vi "ProdaNG.Tree.Proc.Update.vi"(4 "Configuration":T1={"ShowUnreleased"=FALSE, "Param1"="", "ParamStartIdx"=0, "Slots"=1} {"Slots" min=1 max=2; "ParamStartIdx" min=0 max=1}, 6 "VariantFilter":string caption="Wabco Part Filter", 7 "Tree":refnum<vi>, 8 "error in (no error)":errorcluster, 11 "dbHandle in":i32) -> (0 "error out":errorcluster, 3 "dbHandle out":i32)   [LabVIEW 2016]
uses:
  ProdaNG.Configurator.Config.ctl
  ProdaNG.Configurator.Glb.vi
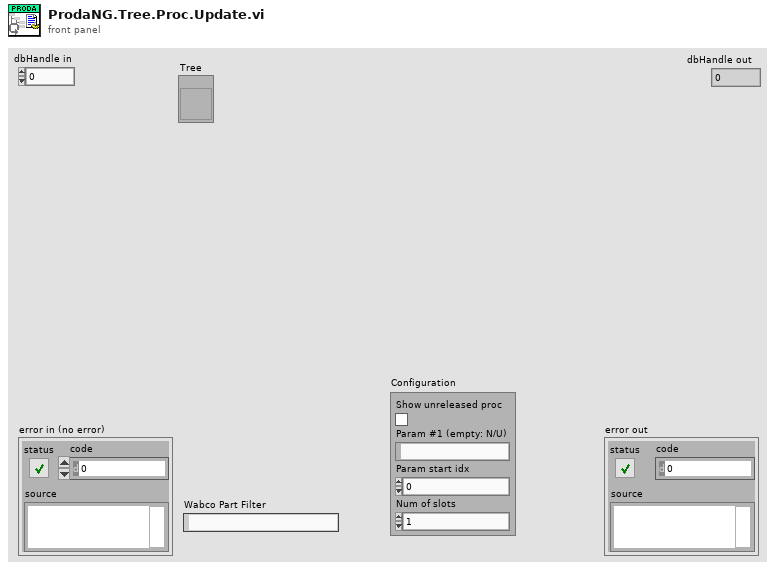
[diagram p1: front panel]
types:
  T1 = typedef "ProdaNG.Configurator.Config.ctl" = cluster{"ShowUnreleased":bool, "Param1":string, "ParamStartIdx":i32, "Slots":i32}
  T2 = cluster{"P_ID":i32, "S_ID":i32, "PS_ID":i32, "WP_ID":i32}
  T3 = typedef "ProdaNG.WabcoPart.ctl" = cluster{"i_id":i32, "workCenterId":i32, "contentId":string, "previewId":string, "mdReason":string, "mdUser":string, "mdTime":string, "productName":string, "wabcoNumber":string}
  T4 = typedef "ProdaNG.Process.ctl" = cluster{"i_id":i32, "productionLineId":i32, "releaseId":i32, "contentId":string, "previewId":string, "mdReason":string, "mdUser":string, "mdTime":string, "description":string}
  T5 = typedef "ProdaNG.ProcessStep.ctl" = cluster{"i_id":i32, "processId":i32, "systemId":i32, "releaseId":i32, "processSequence":i32, "limitYellow":dbl, "limitRed":dbl, "mdReason":string, "mdUser":string, "mdTime":string, "filename":string, "transfer":string, "description":string}
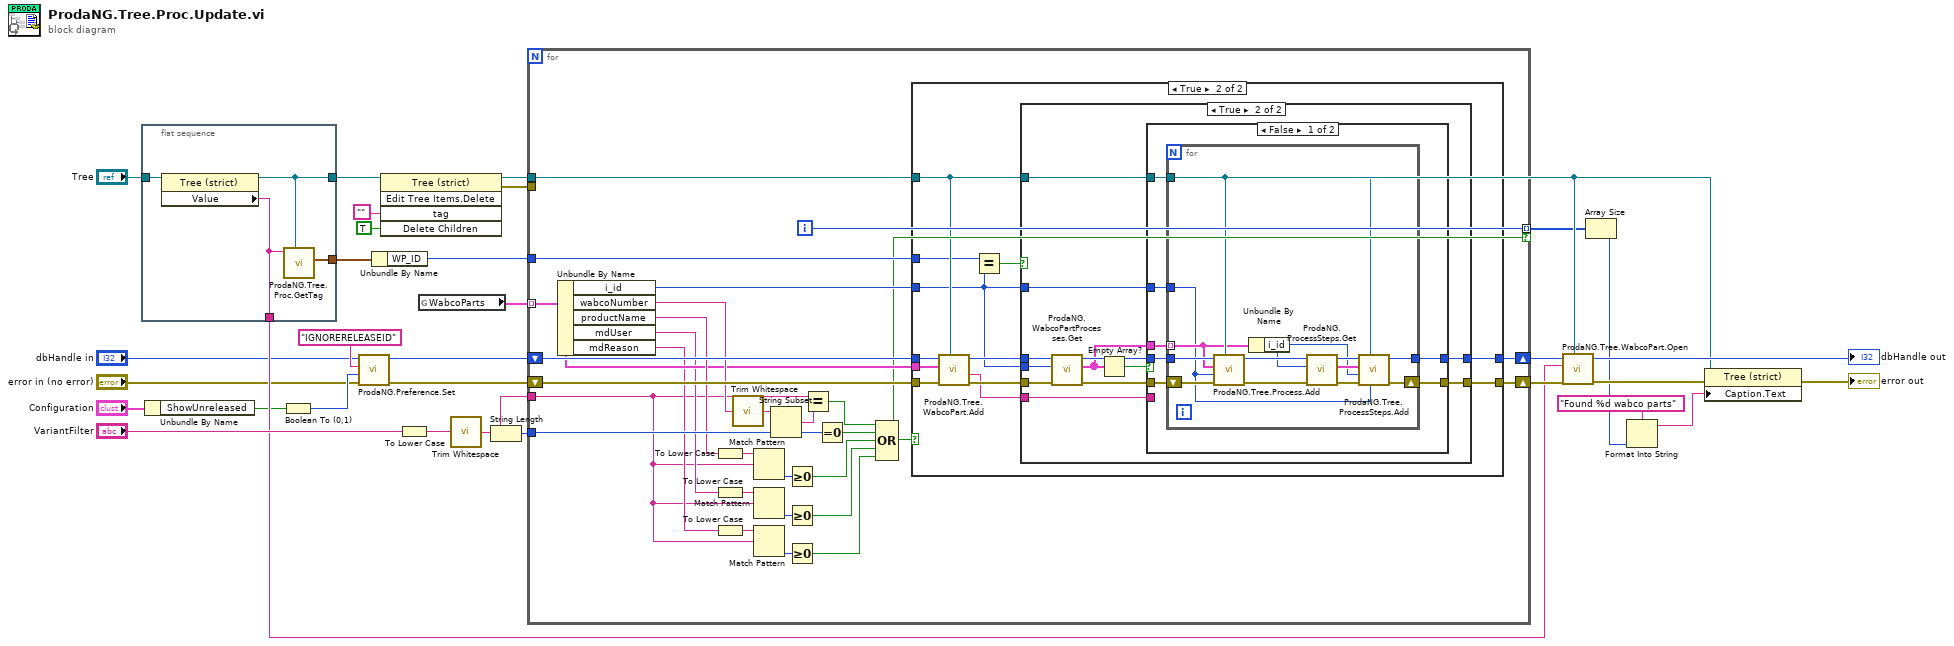
[diagram p0: block diagram]
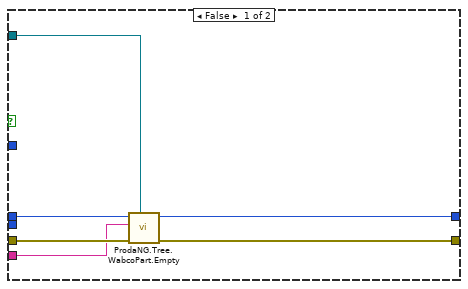
[diagram p3: hidden frame]
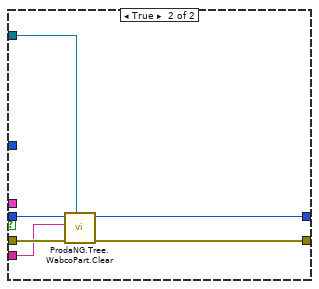
[diagram p4: hidden frame]
diagram:
  n1 = flat-sequence {
    tunnel: "Tree" -> [w34]
    tunnel: [w33] -> w24
    tunnel: [w32] -> w23
    tunnel: [w31] -> w20
    frame #0 {
      n2 = property class="Tree (strict)"(reference=w34) -> (reference out=w33:refnum<vi>, "Value"=w31:string)  [unwired: 1 in, 1 out]
      n3 = call "ProdaNG.Tree.Proc.GetTag.vi"("Tree"=w33, "Tag"=w31) -> ("Identification"=w32:T2)  [unwired: 5 in, 4 out]
    }
  }
  n4 = Unbundle By Name("Configuration") -> ("ShowUnreleased"=w1:bool)
  n5 = Boolean To (0,1)(Boolean=w1) -> (0, 1=w8:i16)
  n6 = call "ProdaNG.Preference.Set.vi"("error in"="error in (no error)", "value"=w8, "key"="IGNORERELEASEID", "dbHandleIn"="dbHandle in") -> ("error out"=w6:errorcluster, "dbHandle"=w5:i32)  [unwired: 6 in]
  n7 = Unbundle By Name(w23) -> ("WP_ID"=w22:i32)
  n8 = invoke class="Tree (strict)" method="Edit Tree Items.Delete"(reference=w24, "tag"="", "Delete Children"=TRUE ("Delete Children?")) -> (reference out=w13:refnum<vi>, error out=w26:errorcluster)  [unwired: 2 in, 3 out]
  n9 = To Lower Case(string="VariantFilter") -> (all lower case string=w17:string)
  n10 = global read "ProdaNG.Configurator.Glb.vi" "WabcoParts"() -> (w16:T3[])
  n11 = call <vilib>:"Trim Whitespace.vi"("string"=w17) -> ("trimmed string"=w18:string)  [unwired: 1 in]
  n12 = String Length(string=w18) -> (length=w19:i32)
  n13 = for {
    shift-right: [w61] -> w30
    shift-left: w5 -> [w62]
    shift-right: [w60] -> w21
    shift-left: w6 -> [w63]
    tunnel: w13 -> [w59]
    tunnel: w26 -> [_]
    tunnel: w22 -> [w58]
    tunnel: w19 -> [w54]
    tunnel: w18 -> [w37]
    tunnel: w16 -> [w49] mode=indexing
    tunnel: [w48] -> w12 mode=indexing if=w47
    i -> [w48]
    n14 = Unbundle By Name(w49) -> ("i_id"=w53:i32, "wabcoNumber"=w57:string, "productName"=w52:string, "mdUser"=w42:string, "mdReason"=w38:string)
    n15 = To Lower Case(string=w52) -> (all lower case string=w50:string)
    n16 = To Lower Case(string=w42) -> (all lower case string=w44:string)
    n17 = To Lower Case(string=w38) -> (all lower case string=w39:string)
    n18 = call <vilib>:"Trim Whitespace.vi"("string"=w57) -> ("trimmed string"=w55:string)  [unwired: 1 in]
    n19 = Match Pattern(string=w50, regular expression=w37) -> (offset past match=w51:i32)  [unwired: 1 in, 3 out]
    n20 = Match Pattern(string=w44, regular expression=w37) -> (offset past match=w43:i32)  [unwired: 1 in, 3 out]
    n21 = Match Pattern(string=w39, regular expression=w37) -> (offset past match=w40:i32)  [unwired: 1 in, 3 out]
    n22 = String Subset(string=w55, length (rest)=w54) -> (substring=w56:string)  [unwired: 1 in]
    n23 = Greater Or Equal To 0?(x=w51) -> (x >= 0?=w41:bool)
    n24 = Greater Or Equal To 0?(x=w43) -> (x >= 0?=w36:bool)
    n25 = Greater Or Equal To 0?(x=w40) -> (x >= 0?=w35:bool)
    n26 = Equal?(x=w37, y=w56) -> (x = y?=w46:bool)
    n27 = Equal To 0?(x=w54) -> (x = 0?=w45:bool)
    n28 = Compound Arithmetic op=OR(w46, w45, w41, w36, w35) -> (w47:bool)
    n29 = case shown="True" w47 {
      tunnel: w63 -> [w64 w73]
      tunnel: w62 -> [w65 w76]
      tunnel: [w65 w75] -> w61
      tunnel: [w64 w74] -> w60
      tunnel: w49 -> [_ w72]
      tunnel: w59 -> [_ w71]
      tunnel: w58 -> [_ w69]
      tunnel: w53 -> [_ w67]
      frame False {
      }
      frame True {
        n30 = call "ProdaNG.Tree.WabcoPart.Add.vi"("Tree"=w71, "error in (no error)"=w73, "WabcoPart"=w72) -> ("error out"=w70:errorcluster, "tag"=w66:string)  [unwired: 7 in]
        n31 = Equal?(x=w69, y=w67) -> (x = y?=w68:bool)
        n32 = case shown="True" w68 {
          tunnel: w76 -> [w81 w93]
          tunnel: [w81 w89] -> w75
          tunnel: [w78 w88] -> w74
          tunnel: w71 -> [w80 w86]
          tunnel: w70 -> [w79 w85]
          tunnel: w67 -> [_ w84]
          tunnel: w67 -> [_ w83]
          tunnel: w66 -> [w77 w82]
          frame False {
            n33 = call "ProdaNG.Tree.WabcoPart.Empty.vi"("Tree"=w80, "error in (no error)"=w79, "Tag"=w77) -> ("error out"=w78:errorcluster)  [unwired: 8 in]
          }
          frame True {
            n34 = call "ProdaNG.WabcoPartProcesses.Get.vi"("error in (no error)"=w85, "WabcoPartId"=w84, "dbHandleIn"=w93) -> ("error out"=w91:errorcluster, "Proc"=w87:T4[], "dbHandle"=w90:i32)  [unwired: 6 in]
            n35 = Empty Array?(array=w87) -> (empty?=w92:bool)
            n36 = case shown="False" w92 {
              tunnel: w91 -> [w95 w115]
              tunnel: w90 -> [w99 w116]
              tunnel: [w98 w116] -> w89
              tunnel: [w97 w112] -> w88
              tunnel: w87 -> [w100 _]
              tunnel: w86 -> [w96 w114]
              tunnel: w83 -> [w94 _]
              tunnel: w82 -> [_ w113]
              frame False {
                n37 = for {
                  tunnel: w99 -> [w111]
                  tunnel: [w104] -> w98
                  tunnel: w100 -> [w102] mode=indexing
                  shift-right: [w105] -> w97
                  shift-left: w95 -> [w109]
                  tunnel: w96 -> [w110]
                  tunnel: w94 -> [w101]
                  n38 = call "ProdaNG.Tree.Process.Add.vi"("Tree"=w110, "error in (no error)"=w109, "WabcoPartId"=w101, "ProcessStep"=w102) -> ("error out"=w108:errorcluster)  [unwired: 7 in]
                  n39 = Unbundle By Name(w102) -> ("i_id"=w103:i32)
                  n40 = call "ProdaNG.ProcessSteps.Get.vi"("error in (no error)"=w108, "processId"=w103, "dbHandleIn"=w111) -> ("error out"=w106:errorcluster, "ProcSteps"=w107:T5[], "dbHandle"=w104:i32)  [unwired: 6 in]
                  n41 = call "ProdaNG.Tree.ProcessSteps.Add.vi"("WabcoPartId"=w101, "Tree"=w110, "error in (no error)"=w106, "ProcId"=w103, "ProcSteps in"=w107) -> ("error out"=w105:errorcluster)  [unwired: 5 in, 1 out]
                }
              }
              frame True {
                n42 = call "ProdaNG.Tree.WabcoPart.Clear.vi"("Tree"=w114, "error in (no error)"=w115, "Tag"=w113) -> ("error out"=w112:errorcluster)  [unwired: 8 in]
              }
            }
          }
        }
      }
    }
  }
  "dbHandle out" <- w30
  n43 = call "ProdaNG.Tree.WabcoPart.Open.vi"("Tree"=w13, "error in (no error)"=w21, "Tag"=w20) -> ("error out"=w15:errorcluster)  [unwired: 8 in]
  n44 = Array Size(array=w12) -> (size(s)=w11:i32)
  n45 = Format Into String(format string="Found %d wabco parts", w11) -> (resulting string=w9:string)  [unwired: 2 in, 1 out]
  n46 = property class="Tree (strict)"(reference=w13, error in=w15, "Caption.Text"=w9) -> (error out=→"error out":errorcluster)  [unwired: 1 out]
